vi "Tune and Beat Learning.vi"() -> ()   [LabVIEW 2025]
uses:
  <vilib>/Platform/TimedLoop/XDataNode/timing_clust.ctl
  <vilib>/Platform/TimedLoop/XDataNode/nitl_modes.ctl
  <vilib>/Platform/TimedLoop/XDataNode/wakeup.ctl
  <vilib>/addons/_NISVFA/_Baseband FFT/SVFA Power Spectrum (1 Ch).vi
  <vilib>/platform/TimedLoop/XDataNode/XDataNode.xnode
  <vilib>/Platform/TimedLoop/XDataNode/XDNodeRunTimeDep.lvlib
  home/lvuser/natinst/piano_note_array.so
  home/lvuser/natinst/drum_synth.so
  home/lvuser/natinst/drum_synth_v2.so
  home/lvuser/natinst/melody_learn_v5.so
panel:
  in  "Mode":enum32{"Sound Desgin"}(tab)
  in  "groove mutation":dbl(slide)=0.10240963855421688 scale=0.0..1.0
  in  "energy":dbl(slide)=0.1566265060240964 scale=0.0..1.0
  in  "notes":i32=15
  in  "style":T1(ring)=enum."Upbeat"
  in  "drum_kit":T2(ring)=enum."Beat Box"
  in  "Like":bool
  out "Spectrum":cluster{"f0":dbl, "df":dbl, "magnitude":dbl[]}(graph)={"f0"=0.0, "df"=10.000016300026568, "magnitude"=[]}
  in  "file path (use dialog)":path=path "/home/lvuser/natinst/training/coeffs_v5_initial.csv"
  in  "Read file":bool
  in  "stop":bool
  in  "Generate":bool
  in  "samples":i32=4410
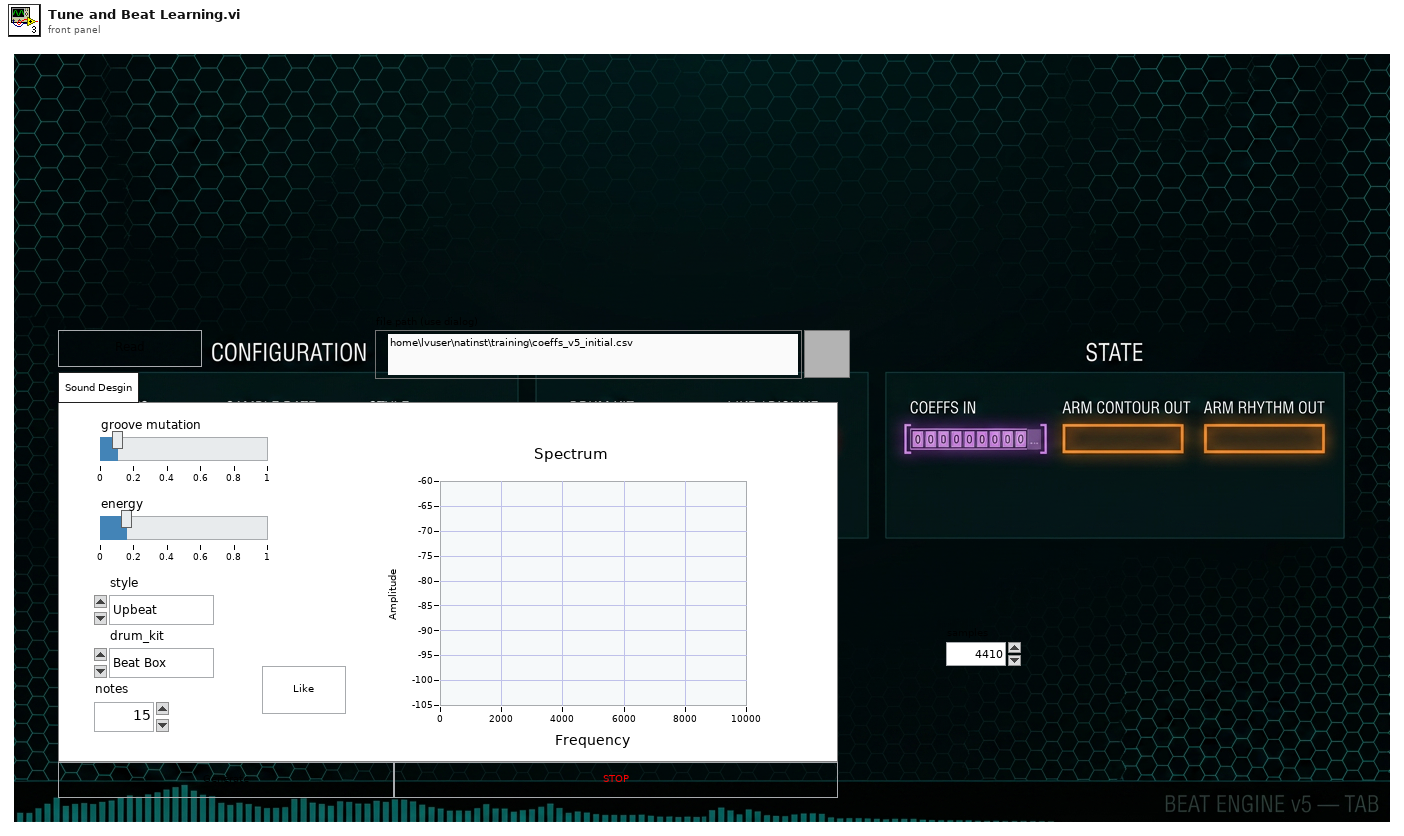
[diagram p1: front panel]
types:
  T1 = enum16{"Lyrical", "Upbeat", "Mixed rythyms", "Jazz", "Rock Band", "Beat"}
  T2 = enum16{"Rock", "Raggae", "Beat Box", "Latin", "Electronic"}
  T3 = typedef "XDNodeRunTimeDep.lvlib/timing_clust.ctl" = cluster{"Expected End [f-1]":u64, "Actual End [f-1]":u64, "Finished Late? [f-1]":bool, "Expected End [i-1]":u64, "Actual End [i-1]":u64, "Finished Late? [i-1]":bool, "Expected Start [i]":u64, "Actual Start [i]":u64, "Expected Start [f]":u64, "Actual Start [f]":u64, "Source Name":string, "Structure Name":string, "Period":i64, "Deadline":i64, "Offset":i64, "Start":i64, "Priority":i32, "Timeout":i32, "Mode":T4, "Wakeup Reason":T5, "Error":errorcluster, "Source Type":string, "Secondary Source Type":string, "Global End Time":u64, "Global Start Time":u64, "Frame Duration":u64, "Iteration Duration":u64, "Assigned CPU":i32, "I/O Scan Engine Mode":u32}
  T4 = typedef "XDNodeRunTimeDep.lvlib/nitl_modes.ctl" = enum32{"No Change", "Process missed periods, maintain original phase", "Discard missed periods, maintain original phase", "Process missed periods, ignore original phase", "Discard missed periods, ignore original phase"}
  T5 = typedef "XDNodeRunTimeDep.lvlib/wakeup.ctl" = enum32{"Normal", "Aborted", "Asynchronous wakeup", "Timing source error", "Timed loop error", "Timeout"}
  T6 = enum16{"open", "replace", "create", "open or create", "replace or create", "replace or create with confirmation"}
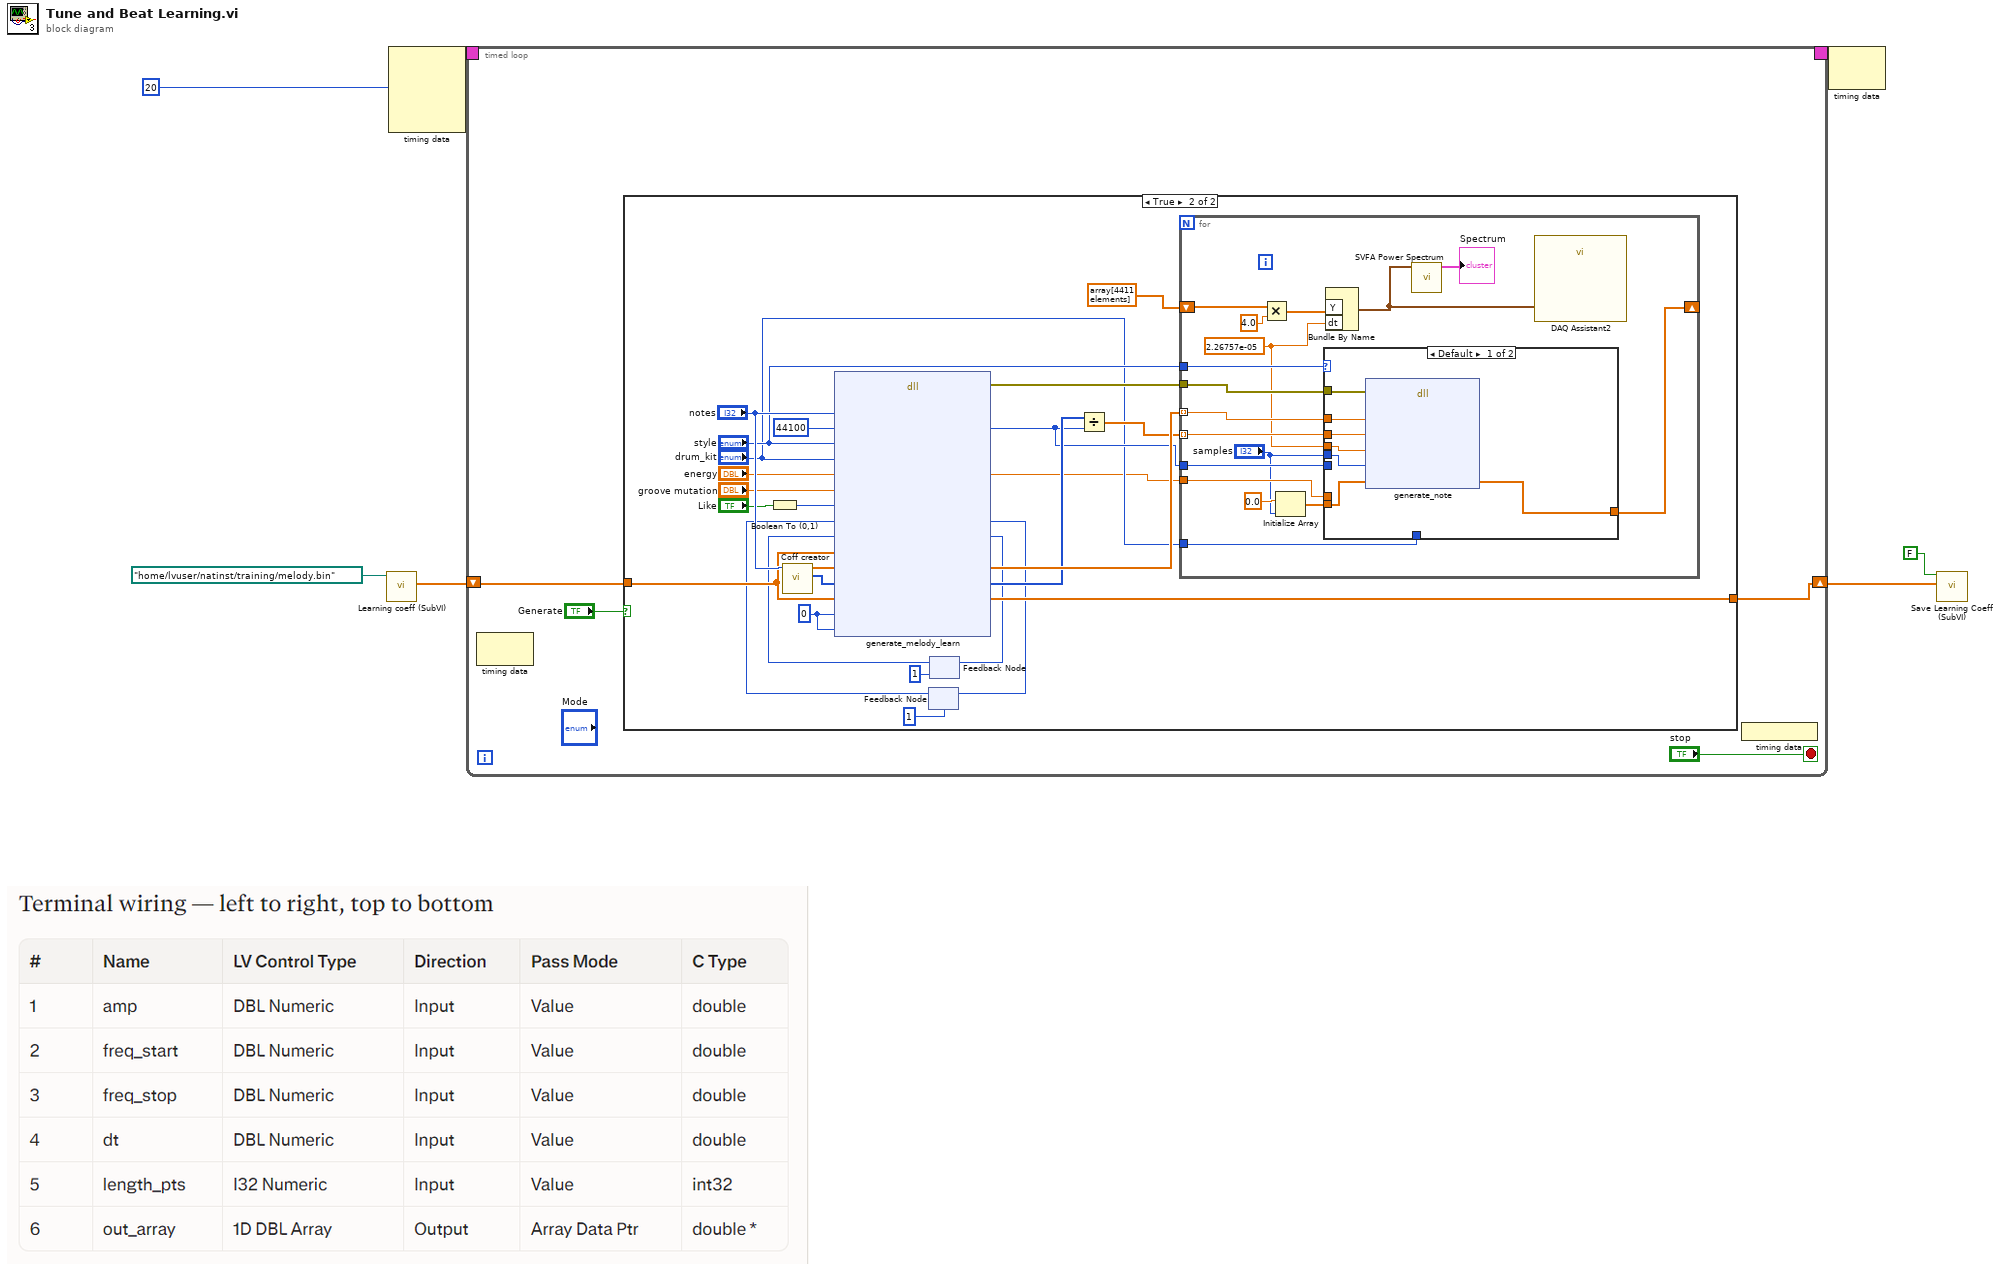
[diagram p0: block diagram]
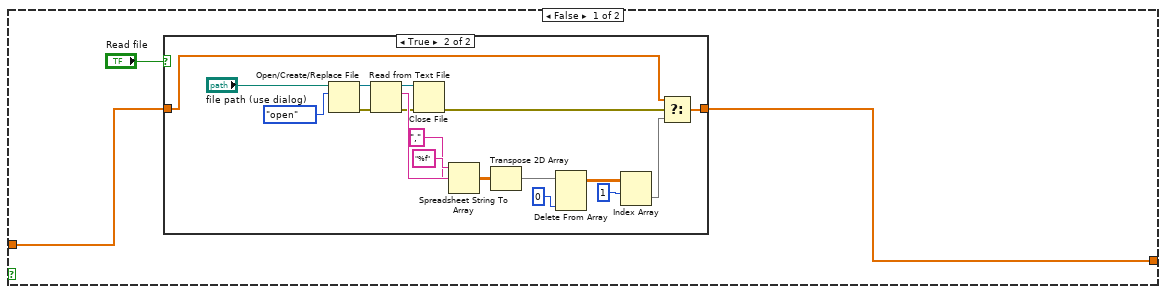
[diagram p2: hidden frame]
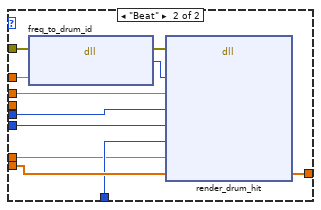
[diagram p4: hidden frame]
diagram:
  n1 = call "Learning coeff (SubVI).vi"("file path (use dialog)"=path "/home/lvuser/natinst/training/melody.bin") -> ("initialized array"=w2:dbl[])  [unwired: 9 in, 1 out]
  n2 = node-c288(i64 20 ("Period")) -> (w7:T3)  [unwired: 3 in]
  n3 = timed-loop {
    timing: w7 -> [_]
    timing-out: [_] -> w6
    shift-right: [w10] -> w3
    shift-left: w2 -> [w8]
    stop <- "stop" stop-if-true
    n4 = node-c288() -> ()  [unwired: 1 in, 1 out]
    n5 = case shown="True" "Generate" {
      tunnel: [w12 w46] -> w10
      tunnel: w8 -> [w13 w47]
      frame False {
        n6 = case shown="True" "Read file" {
          tunnel: w13 -> [w15 w24]
          tunnel: [w15 w31] -> w12
          frame False {
          }
          frame True {
            n7 = Open/Create/Replace File(file path (use dialog)="file path (use dialog)", operation (0:open)=T6."open") -> (refnum out=w29:refnum<file>, error out=w30:errorcluster)  [unwired: 4 in, 1 out]
            n8 = Read from Text File(file (use dialog)=w29, error in=w30) -> (refnum out=w22:refnum<file>, text=w28:string, error out=w25:errorcluster)  [unwired: 2 in, 1 out]
            n9 = Close File(refnum=w22, error in=w25) -> (error out=w19:errorcluster)  [unwired: 1 out]
            n10 = Spreadsheet String To Array(delimiter (Tab)=",", format string="%f", spreadsheet string=w28) -> (array=w23:dbl[][])  [unwired: 1 in]
            n11 = Transpose 2D Array(2D array=w23) -> (transposed array=w21:dbl[][])
            n12 = Delete From Array(array=w21, index (col)=0 ("index (row)")) -> (array with subset deleted=w17:dbl[][])  [unwired: 2 in, 1 out]
            n13 = Index Array(array=w17, index (row)=1) -> (element=w20:dbl[])  [unwired: 1 in]
            n14 = Select(t=w24, s=w19, f=w20) -> (s? t:f=w31:dbl[])
          }
        }
      }
      frame True {
        w41 = 0
        w44 = 44100
        n15 = Boolean To (0,1)(Boolean="Like") -> (0, 1=w48:i16)
        n16 = call "Coff creator.vi"("notes"="notes") -> ("Array"=w51:i32[], "Array 2"=w56:dbl[])  [unwired: 9 in]
        n17 = feedback #1(1 ("last_arm_rythm")) -> (w34:i32)
        n18 = feedback #2(1 ("last_arm_rythm")) -> (w38:i32)
        n19 = dll-call lib="home/lvuser/natinst/melody_learn_v5.so" fn="generate_melody_learn"("n_notes"="notes", "sample_rate"=w44, "style"="style", "drum_kit"="drum_kit", "energy"="energy", "groove_mutation"="groove mutation", "like_dislike"=w48, "last_arm_contour"=w34, "last_arm_rythm"=w38, "coeffs_in"=w47, "freq_out"=w56, "durs"=w51, "coeff_out"=w47, "arm_countour_out"=w41, "arm_rythym_out"=w41) -> (error out=w53:errorcluster, "last_arm_contour"=w37:i32, "last_arm_rythm"=w39:i32, "freq_out"=w57:dbl[], "durs"=w55:i32[], "coeff_out"=w46:dbl[])  [unwired: 14 in, 1 out]
        n20 = feedback-in #1(w37) -> ()
        n21 = feedback-in #2(w39) -> ()
        n22 = Divide(x=w55, y=w44) -> (x/y=w54:dbl[])
        n23 = for {
          tunnel: w57 -> [w72] mode=indexing
          tunnel: w54 -> [w71] mode=indexing
          tunnel: w53 -> [w70]
          shift-right: [w61] -> _
          shift-left: dbl[] array[4411 elements] ("out") -> [w58]
          tunnel: "style" -> [w69]
          tunnel: w44 -> [w68]
          tunnel: "drum_kit" -> [w67]
          tunnel: "energy" -> [w66]
          w62 = 2.26757e-05 ("dt")
          n24 = Multiply(x=w58, y=4.0) -> (x*y=w59:dbl[])
          n25 = Initialize Array(0.0 ("velocity"), "samples") -> (w74:dbl[])
          n26 = case shown="Default" w69 {
            tunnel: "samples" -> [w81 w92]
            tunnel: w74 -> [w80 w91]
            tunnel: w62 -> [w79 _]
            tunnel: w72 -> [w78 w87]
            tunnel: w71 -> [w77 w90]
            tunnel: w70 -> [w76 w85]
            tunnel: [w75 w89] -> w61
            tunnel: w68 -> [_ w88]
            tunnel: w67 -> [_ w83]
            tunnel: w66 -> [_ w82]
            frame Default {
              n27 = dll-call lib="home/lvuser/natinst/piano_note_array.so" fn="generate_note"(error in=w76, "freq"=w78, "velocity"=w77, "dt"=w79, "n_samples"=w81, "out"=w80) -> ("out"=w75:dbl[])  [unwired: 7 in, 2 out]
            }
            frame "Beat" {
              n28 = dll-call lib="home/lvuser/natinst/drum_synth.so" fn="freq_to_drum_id"(error in=w85, "freq"=w87) -> (error out=w86:errorcluster, "return type"=w84:i32)  [unwired: 3 in, 1 out]
              n29 = dll-call lib="home/lvuser/natinst/drum_synth_v2.so" fn="render_drum_hit"(error in=w86, "drum_id"=w84, "velocity"=w90, "n_samples"=w92, "sample_rate"=w88, "drum_kit"=w83, "energy"=w82, "out"=w91) -> ("out"=w89:dbl[])  [unwired: 9 in, 2 out]
            }
          }
          n30 = Bundle By Name("Y"=w59, "dt"=w62) -> (w65:waveform(dbl))  [unwired: 1 in]
          n31 = call-poly <vilib>:"SVFA Power Spectrum.vi"("scaled signal [EU]"=w65) -> ("power spectrum [dB EU]"=→"Spectrum":cluster{"f0":dbl, "df":dbl, "magnitude":dbl[]})  [unwired: 13 in, 5 out]
          n32 = call "DAQ Assistant2"("data"=w65) -> ()  [unwired: 17 in, 2 out]
        }
      }
    }
    n33 = node-c288() -> ()  [unwired: 1 out]
  }
  n34 = node-c288(w6) -> ()  [unwired: 1 out]
  n35 = call "Save Learning Coeff (SubVI).vi"("initialized array"=w3, "Boolean"=FALSE) -> ()  [unwired: 10 in]
